vi "UndefineCustomCode.vi"(9 "Error in":errorcluster caption="Error in (no error)", 11 "Custom code":i32) -> ()   [LabVIEW 2017, in "GPError.lvlib"]
doc: "Deletes any prior definition(s) of <B>Custom code</B> made with the DefineCustomCode function.\n\nThis VI is inlined and it runs only if there is no error on <B>Error in</B>.\n\nSteen Schmidt\nGPower\n17/7 2013"
uses:
  GPError.lvlib
  FG/CustomErrorFGFunction.ctl
panel:
  # "Copyright © 2013\nSteen Schmidt, GPower\nSee enclosed license file for terms and conditions"
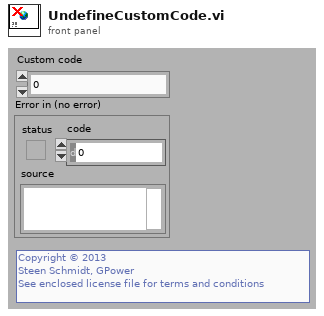
[diagram p1: front panel]
types:
  T1 = typedef "GPError.lvlib/CustomErrorFGFunction.ctl" = enum16{"Get custom descriptions", "Set custom code", "Unset custom code"}
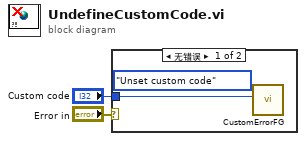
[diagram p0: block diagram]
diagram:
  n1 = case shown="无错误" "Error in" {
    tunnel: "Custom code" -> [w3 _]
    frame No Error {
      n2 = call "CustomErrorFG.vi"("Custom code"=w3, "Function"=CustomErrorFGFunction."Unset custom code") -> ()  [unwired: 8 in, 2 out]
    }
    frame Error {
    }
  }
